vi "GetText.vi"(8 "error in (no error)":errorcluster, 11 "Markdown in":refnum<class "Markdown.lvclass">) -> (0 "error out":errorcluster, 2 "Text":string, 3 "Markdown out":refnum<class "Markdown.lvclass">)   [LabVIEW 2021, in "LvMarkdown.lvlib" / "Markdown.lvclass"]
uses:
  Markdown.lvclass
  Markdown.lvclass/Markdown.ctl
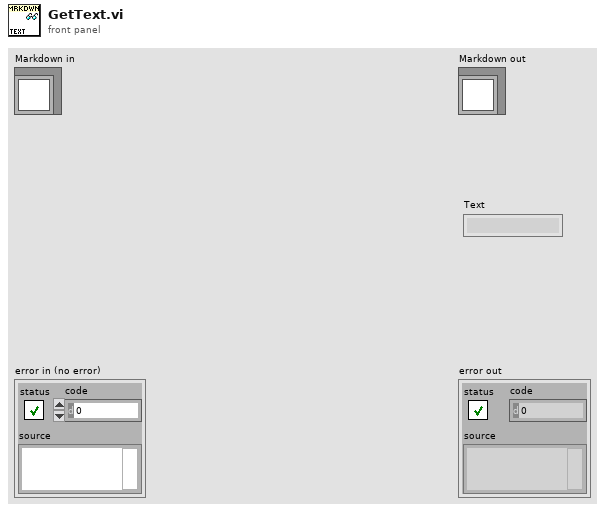
[diagram p1: front panel]
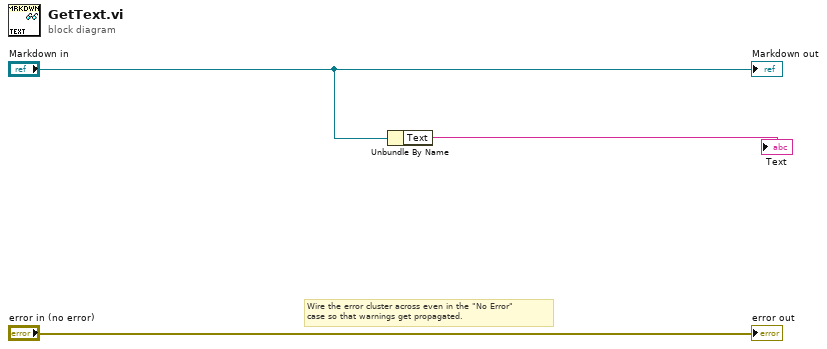
[diagram p0: block diagram]
diagram:
  # "Wire the error cluster across even in the \"No Error\"\ncase so that warnings get propagated."
  n1 = Unbundle By Name("Markdown in") -> ("Text"=→"Text":string)
  "error out" <- "error in (no error)"
  "Markdown out" <- "Markdown in"
